vi "Wait On Execution.vi"(8 "error in (no error)":errorcluster, 11 "Synchronous Write Callback in":refnum<class "Synchronous Write Callback.lvclass">) -> (0 "error out":errorcluster)   [LabVIEW 2020, in "Network Messenger.lvlib" / "Synchronous Write Callback.lvclass"]
uses:
  <vilib>/gpm_packages/@cs/Network-interface/Source/Network Messenger/Synchronous Write Callback/Synchronous Write Callback.lvclass
  <vilib>/gpm_packages/@cs/Network-interface/Source/Network Messenger/Synchronous Write Callback/Synchronous Write Callback.lvclass/Synchronous Write Callback.ctl
  <vilib>/ErrorRing/Error Ring.xnode
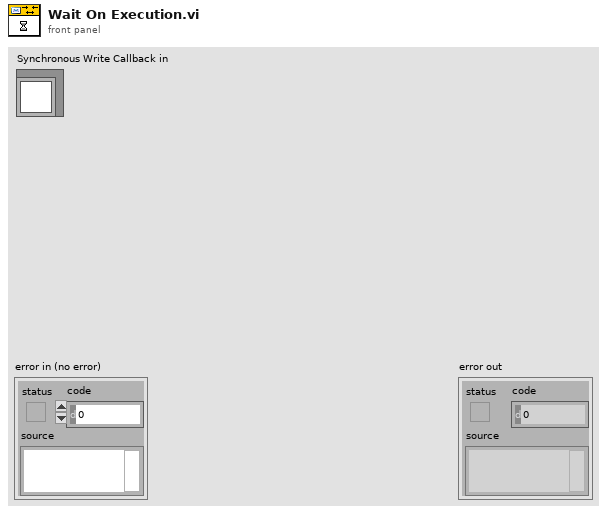
[diagram p1: front panel]
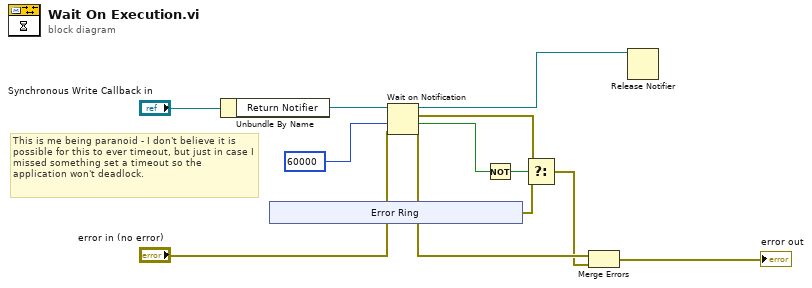
[diagram p0: block diagram]
diagram:
  # "This is me being paranoid - I don't believe it is possible for this to ever timeout, but just in case I missed something set a timeout so the application won't deadlock."
  n1 = Unbundle By Name("Synchronous Write Callback in") -> ("Return Notifier"=w11:refnum<notifier>)
  n2 = xnode "Error Ring"() -> ("error out"=w2:errorcluster)
  n3 = Wait on Notification(notifier=w11, timeout in ms (-1)=60000, error in (no error)="error in (no error)") -> (notifier out=w1:refnum<notifier>, notification=w7:errorcluster, timed out?=w9:bool, error out=w6:errorcluster)  [unwired: 1 in]
  n4 = Not(x=w9) -> (.not. x?=w8:bool)
  n5 = Select(t=w7, s=w8, f=w2) -> (s? t:f=w5:errorcluster)
  n6 = Merge Errors(w6, w5) -> (→"error out":errorcluster)
  n7 = Release Notifier(notifier=w1) -> ()  [unwired: 2 in, 3 out]
